vi "Initialize Conditional Expression.vi"(8 "error in (no error)":errorcluster, 10 "Expression string":string, 11 "Output Sequencer in":refnum<class "Output Sequencer.lvclass">) -> (0 "error out":errorcluster, 2 "Expression Data":T1, 3 "Output Sequencer out":refnum<class "Output Sequencer.lvclass">)   [LabVIEW 2024, in "Output Sequencer.lvlib" / "Output Sequencer.lvclass"]
uses:
  Output Sequencer.lvclass
  Types/Expression Data.ctl
  <vilib>/LAVA/muParser/mupExpr/mupExpr.lvclass
  Output Sequencer.lvclass/Output Sequencer.ctl
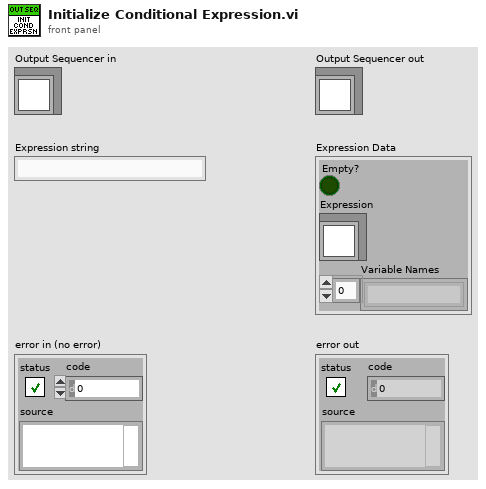
[diagram p1: front panel]
types:
  T1 = typedef "Output Sequencer.lvlib/Output Sequencer.lvclass/Expression Data.ctl" = cluster{"Empty?":bool, "Expression":refnum<class "mupExpr.lvclass">, "Variable Names":string[]}
  T2 = cluster{"error code":i32, "error message":string, "error pos":i32, "error token":string}
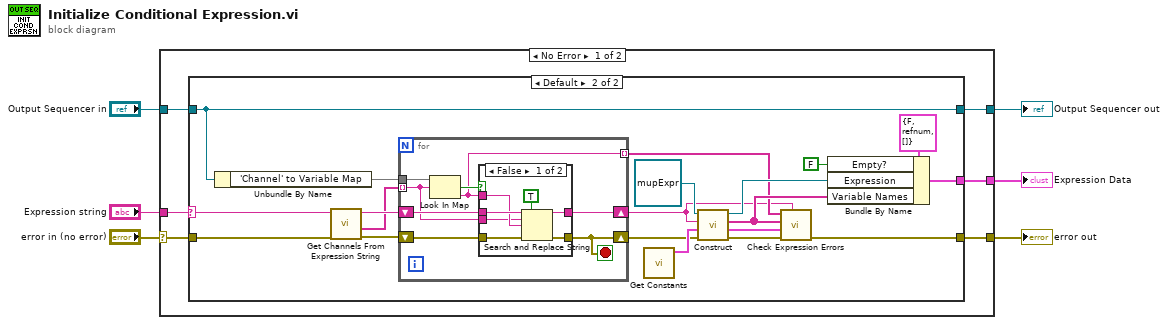
[diagram p0: block diagram]
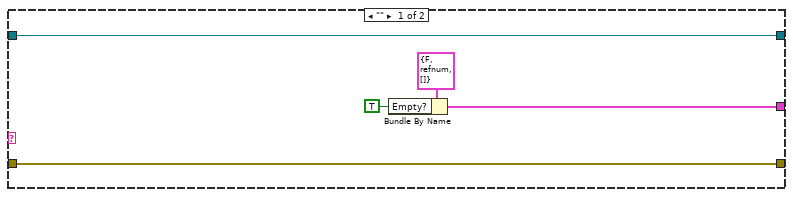
[diagram p2: hidden frame]
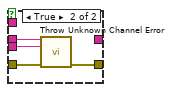
[diagram p3: hidden frame]
diagram:
  n1 = case shown="No Error" "error in (no error)" {
    selector: "error in (no error)" -> [w7 w58]
    tunnel: [w12 _] -> w6
    tunnel: "Expression string" -> [w11 _]
    tunnel: [w10 w58] -> w4
    tunnel: "Output Sequencer in" -> [w9 w57]
    tunnel: [w8 w57] -> w2
    frame No Error {
      n2 = case shown="Default" w11 {
        selector: w11 -> [_ w25]
        tunnel: w9 -> [w13 w26]
        tunnel: w7 -> [w14 w31]
        tunnel: [w14 w18] -> w10
        tunnel: [w16 w28] -> w12
        tunnel: [w13 w26] -> w8
        frame "" {
          n3 = Bundle By Name(cluster=T1 {"Empty?"=FALSE, "Expression"=refnum, "Variable Names"=[]} ("Expression Data"), "Empty?"=TRUE) -> (w16:T1)
        }
        frame Default {
          n4 = Unbundle By Name(w26) -> ("'Channel' to Variable Map"=w33:map{string, string})
          n5 = call "Get Channels From Expression String.vi"("error in (no error)"=w31, "Expression String in"=w25) -> ("error out"=w30:errorcluster, "Channels (with quotes)"=w24:string[], "Expression String out"=w32:string)  [unwired: 6 in, 1 out]
          n6 = for {
            tunnel: w24 -> [w41] mode=indexing
            tunnel: w33 -> [w45]
            shift-right: [w39] -> w29
            shift-left: w30 -> [w44]
            shift-right: [w40] -> w19
            shift-left: w32 -> [w42]
            tunnel: [w38] -> w20 mode=indexing
            stop <- w39 stop-if-true
            n7 = Look In Map(map=w45, key=w41) -> (key not found?=w43:bool, value=w38:string)  [unwired: 1 in]
            n8 = case shown="False" w43 {
              tunnel: w44 -> [w51 w54]
              tunnel: [w50 w53] -> w39
              tunnel: w38 -> [w48 _]
              tunnel: w42 -> [w49 w55]
              tunnel: w41 -> [w47 w56]
              tunnel: [w46 _] -> w40
              frame False {
                n9 = Search and Replace String(replace all?=TRUE ("replace all? (F)"), input string=w49, search string=w47, replace string=w48, error in=w51) -> (result string=w46:string, error out=w50:errorcluster)  [unwired: 3 in, 2 out]
              }
              frame True {
                n10 = call "Throw Unknown Channel Error.vi"("error in (no error)"=w54, "Missing Channel"=w56, "Expression String in"=w55) -> ("error out"=w53:errorcluster)  [unwired: 8 in]
              }
            }
          }
          n11 = call "Get Constants.vi"() -> ("Constants"=w34:cluster{"name":string, "value":dbl}[])  [unwired: 11 in]
          n12 = call-dynamic "Construct.vi"("error in (no error)"=w29, "Constants"=w34, "Expression"=w19, "muExpr in"=refnum<class "mupExpr.lvclass"> refnum) -> ("error out"=w23:errorcluster, "error details"=w22:T2, "Variable Names"=w21:string[], "mupExpr out"=w37:refnum<class "mupExpr.lvclass">)  [unwired: 4 in]
          n13 = call "Check Expression Errors.vi"("Expression String in"=w19, "error in (no error)"=w23, "Parser Error Details"=w22, "Found Variables"=w21, "Expected Variables"=w20) -> ("error out"=w18:errorcluster)  [unwired: 6 in]
          n14 = Bundle By Name(cluster=T1 {"Empty?"=FALSE, "Expression"=refnum, "Variable Names"=[]} ("Expression Data"), "Empty?"=FALSE, "Expression"=w37, "Variable Names"=w21) -> (w28:T1)
        }
      }
    }
    frame Error {
    }
  }
  "Expression Data" <- w6
  "error out" <- w4
  "Output Sequencer out" <- w2
